vi "EllipRegionConstraint_getMaxVelocity.vi"(8 "Velocity":dbl, 9 "Curvature":dbl, 10 "statePose":T4={"TRANSLATION"={"X"=0.0, "Y"=0.0}, "ROTATION"={"VALUE"=0.0, "COS"=1.0, "SIN"=0.0}} {"ROTATION"."SIN" format="%13.4f"; "ROTATION"."COS" format="%13.4f"; "ROTATION"."VALUE" format="%13.4f"; "TRANSLATION"."Y" format="%14.3f"; "TRANSLATION"."X" format="%14.3f"}, 11 "ELLIP_REGION_CONSTRAINT":T1={"Center"={"X"=0.0, "Y"=0.0}, "Radii"={"X"=0.0, "Y"=0.0}, "Constraint"=variant, "Constraint Type"=enum."DIFF DRIVE KINEMATICS", "IM UNIQUE"=FALSE} {"Radii"."Y" format="%14.3f"; "Radii"."X" format="%14.3f"; "Center"."Y" format="%14.3f"; "Center"."X" format="%14.3f"}) -> (3 "absMaxVelocity":dbl)   [LabVIEW 2019, in "Trajectory_Library.lvlib"]
doc: "Return the maximum allowed velocity given the provided conditions.\n\nEnsure each individual normalized wheel speed is within the defined maximum velocity.\n\nParameters:\n - EllipRegionConstraint - Constraint data structure\n - statePose - current traj state Pose\n - curvature - current traj curvature\n - maxVelocity - current traj max velocity\n\nReturns\n - maxVelocity - Maximum allowed velocity."
uses:
  Trajectory_Library.lvlib
  TypeDef/TRANSLATION2D.ctl
  TypeDef/ROTATION2D.ctl
  TypeDef/POSE2D.ctl
  Enum/TRAJ_CONSTRAINT_TYPES_ENUM.ctl
  TypeDef/TRAJ_CONSTRAINT_ELLIP_REGION.ctl
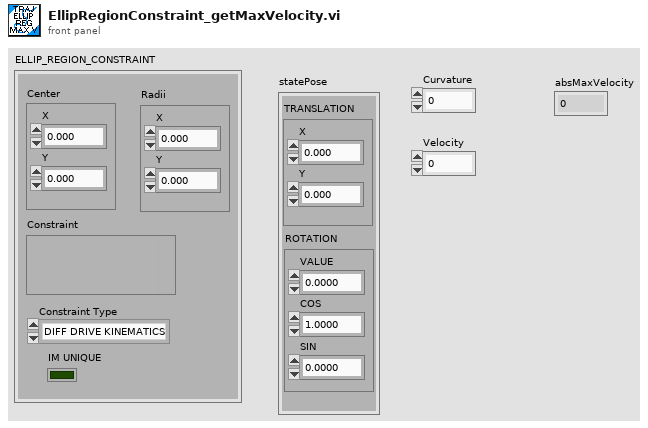
[diagram p1: front panel]
types:
  T1 = typedef "Trajectory_Library.lvlib/TRAJ_CONSTRAINT_ELLIP_REGION.ctl" = cluster{"Center":T2, "Radii":T2, "Constraint":variant, "Constraint Type":T3, "IM UNIQUE":bool}
  T2 = typedef "Trajectory_Library.lvlib/TRANSLATION2D.ctl" = cluster{"X":dbl, "Y":dbl}
  T3 = typedef "Trajectory_Library.lvlib/TRAJ_CONSTRAINT_TYPES_ENUM.ctl" = enum16{"UNDEFINED", "DIFF DRIVE KINEMATICS", "DIFF DRIVE VOLTAGE", "CENTRIPITAL ACCEL", "MECA DRIVE KINEMATICS", "SWERVE DRIVE KINEMATICS", "MAXIMUM VELOCITY", "ELLIPTICAL REGION", "RECTANGULAR REGION"}
  T4 = typedef "Trajectory_Library.lvlib/POSE2D.ctl" = cluster{"TRANSLATION":T2, "ROTATION":T5}
  T5 = typedef "Trajectory_Library.lvlib/ROTATION2D.ctl" = cluster{"VALUE":dbl, "COS":dbl, "SIN":dbl}
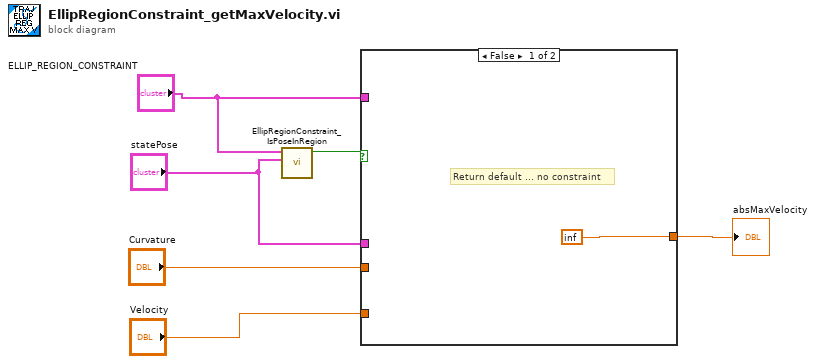
[diagram p0: block diagram]
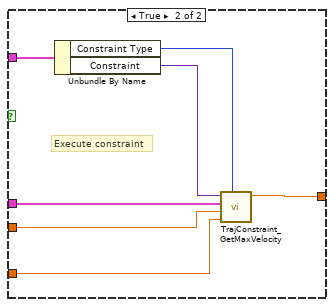
[diagram p2: hidden frame]
diagram:
  n1 = call "EllipRegionConstraint_IsPoseInRegion.vi"("statePose"="statePose", "ELLIP_REGION_CONSTRAINT"="ELLIP_REGION_CONSTRAINT") -> ("PoseInRegion"=w6:bool)  [unwired: 9 in]
  n2 = case shown="False" w6 {
    tunnel: [inf w14] -> w5
    tunnel: "ELLIP_REGION_CONSTRAINT" -> [_ w13]
    tunnel: "statePose" -> [_ w10]
    tunnel: "Curvature" -> [_ w9]
    tunnel: "Velocity" -> [_ w8]
    frame False {
      # "Return default ... no constraint"
    }
    frame True {
      # "Execute constraint"
      n3 = Unbundle By Name(w13) -> ("Constraint Type"=w12:T3, "Constraint"=w11:variant)
      n4 = call "TrajConstraint_GetMaxVelocity.vi"("TrajjectoryConstraintType"=w12, "Velocity"=w8, "Curvature"=w9, "Pose"=w10, "Trajectory Constraint"=w11) -> ("AbsMaxVelocity"=w14:dbl)  [unwired: 5 in, 1 out]
    }
  }
  "absMaxVelocity" <- w5
